vi "StartMoveToPosition.vi"(4 "Go to home":bool, 6 "Polarization":u16(ring) items=["Vertical", "Horizontal"], 8 "error in (no error)":errorcluster, 9 "Position (Antenna or Raster)":i32, 10 "Positions":T1[](array[typedef]), 11 "VXMMotionManager in":refnum<class "VXMMotionManager.lvclass">) -> (0 "error out":errorcluster, 3 "VXMMotionManager out":refnum<class "VXMMotionManager.lvclass">)   [LabVIEW 2018, in "VXMMotionManager.lvclass"]
doc: "convert position 1 - 16 to an X,Y,Z,T position using the \"Position Array\" lookup table."
uses:
  VXMMotionManager.lvclass
  APARMainSubvis/VXM Public API/singleAxisMoveDef.ctl
  APARMainSubvis/VXM Public API/mmWaveAxis.ctl
  MoveAllAbsoluteStates.ctl
  MotionTypes.ctl
  VXMMotionManager.lvclass/VXMMotionManager.ctl
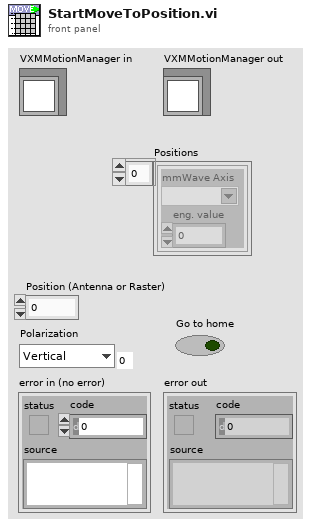
[diagram p1: front panel]
types:
  T1 = typedef "singleAxisMoveDef.ctl" = cluster{"mmWave Axis":T2, "eng. value":dbl}
  T2 = typedef "mmWaveAxis.ctl" = string
  T3 = typedef "MotionTypes.ctl" = enum16{"Homing", "AllAbsolute", "AllHome", "Position", "OneAxisHome", "Clear"}
  T4 = typedef "VXMMotionManager.lvclass/MoveAllAbsoluteStates.ctl" = enum16{"start next move", "wait motion end"}
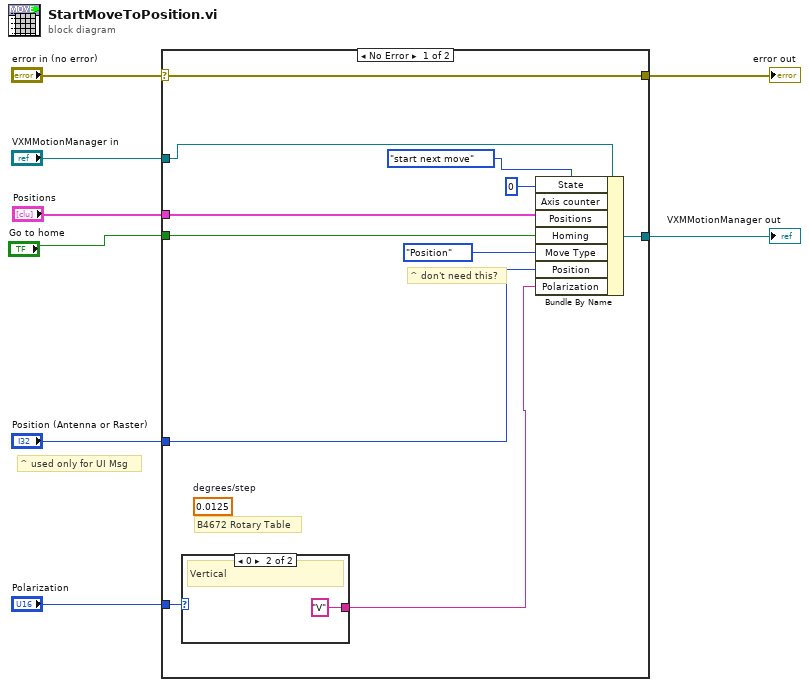
[diagram p0: block diagram]
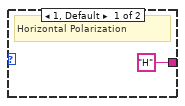
[diagram p2: hidden frame]
diagram:
  # "^ used only for UI Msg"
  n1 = case shown="No Error" "error in (no error)" {
    selector: "error in (no error)" -> [w18 w23]
    tunnel: [w18 w23] -> w7
    tunnel: [w19 w22] -> w5
    tunnel: "VXMMotionManager in" -> [w17 w22]
    tunnel: "Polarization" -> [w16 _]
    tunnel: "Position (Antenna or Raster)" -> [w11 _]
    tunnel: "Positions" -> [w10 _]
    tunnel: "Go to home" -> [w9 _]
    frame No Error {
      (unwired) 0.0125  # degrees/step
      # "^ don't need this?"
      # "B4672 Rotary Table"
      n2 = case shown="0" w16 {
        tunnel: ["H" "V"] -> w12
        frame 1, Default {
          # "Horizontal Polarization"
        }
        frame 0 {
          # "Vertical"
        }
      }
      n3 = Bundle By Name(cluster=w17, "State"=MoveAllAbsoluteStates."start next move", "Axis counter"=0 ("Axis (0-3)"), "Positions"=w10, "Homing"=w9, "Move Type"=MotionTypes."Position", "Position"=w11, "Polarization"=w12) -> (w19:refnum<class "VXMMotionManager.lvclass">)
    }
    frame Error {
    }
  }
  "error out" <- w7
  "VXMMotionManager out" <- w5
